vi "08 Strings.vi"() -> ()   [LabVIEW 2019]
panel:
  out "after ' or : or space":string
  in  "String":string="Fred bought 3 sheep at $10.35 per sheep"
  in  "Info":string="Fred bought 3 sheep at $10.35 per sheep"
  out "cost":dbl
  out "sheep":i32
  out "Smart Replace":string
  out "Replace":string
  out "Option 2":string
  out "Last name first":string
  in  "Name":string="Walker Wind"
  # "Type in your full name (first space last) and hit the Run arrow and see the code execute"
  # "Hit Cmd E to see the diagram (code)"
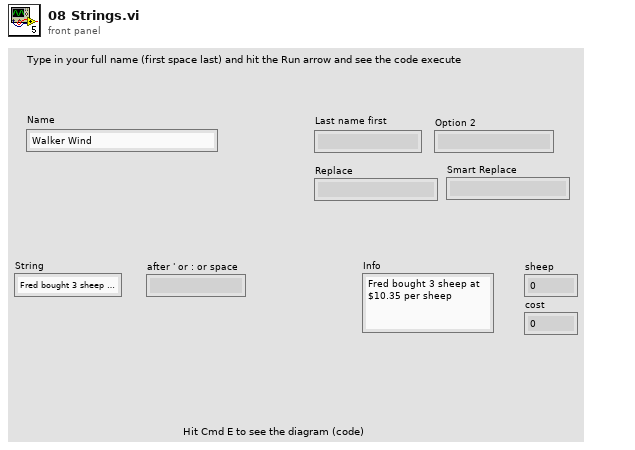
[diagram p1: front panel]
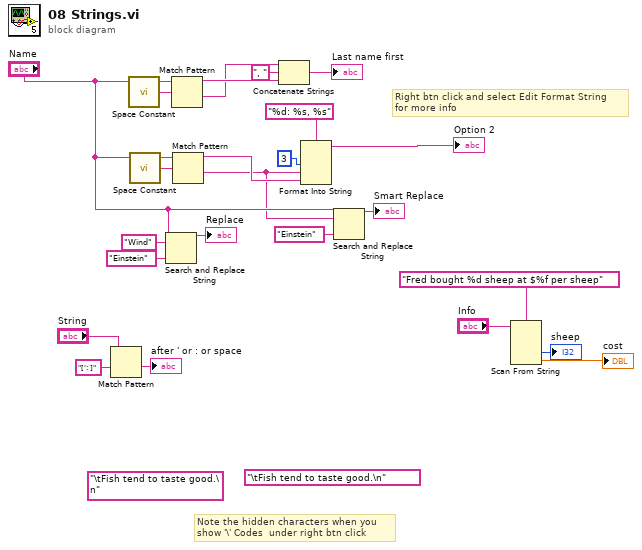
[diagram p0: block diagram]
diagram:
  (unwired) "\tFish tend to taste good.\n" ("regular expression")
  (unwired) "\tFish tend to taste good.\n" ("regular expression")
  # "Note the hidden characters when you\nshow '\\' Codes  under right btn click"
  # "Right btn click and select Edit Format String\nfor more info"
  n1 = Match Pattern(string="String", regular expression="[': ]") -> (after substring=→"after ' or : or space":string)  [unwired: 1 in, 3 out]
  n2 = call <vilib>:"Space Constant.vi"() -> ("String"=w24:string)
  n3 = call <vilib>:"Space Constant.vi"() -> ("String"=w18:string)
  n4 = Search and Replace String(input string="Name", search string="Wind", replace string="Einstein" ("replace string (\"\")")) -> (result string=→"Replace":string)  [unwired: 5 in, 3 out]
  n5 = Match Pattern(string="Name", regular expression=w24) -> (before substring=w23:string, after substring=w22:string)  [unwired: 1 in, 2 out]
  n6 = Match Pattern(string="Name", regular expression=w18) -> (before substring=w17:string, after substring=w8:string)  [unwired: 1 in, 2 out]
  n7 = Concatenate Strings(w22, ", " ("string"), w23) -> (→"Last name first":string)
  n8 = Format Into String(format string="%d: %s, %s", 3 ("input 1"), w8, w17) -> (resulting string=→"Option 2":string)  [unwired: 2 in, 1 out]
  n9 = Search and Replace String(input string="Name", search string=w8, replace string="Einstein" ("replace string (\"\")")) -> (result string=→"Smart Replace":string)  [unwired: 5 in, 3 out]
  n10 = Scan From String(format string="Fred bought %d sheep at $%f per sheep", input string="Info") -> (output 1=→"sheep":i32, output 2=→"cost":dbl)  [unwired: 4 in, 3 out]
